vi "configureHWIO_3_statusBusy.vi"(0 "Camera in":refnum<class "Camera.lvclass">, 1 "on":bool=TRUE, 2 "polarity":u16(ring)=1 items=["high level"=1, "low level"=2], 3 "signal_type":u32(ring) items=["Status Busy", "Status Expos", "Status Line", "Status Armed"], 5 "error in (no error)":errorcluster) -> (14 "Camera out":refnum<class "Camera.lvclass">, 19 "error out":errorcluster)   [LabVIEW 2019, in "Camera.lvclass"]
doc: "Configures HWIO 3 status busy for polarity and status (enabled / disabled), and also fuction (exposure or line). Generates an error if camera is recording or if HWIO configuration is not supported."
uses:
  Camera.lvclass
  pco.sdk/CameraDescription/CameraDescription.lvlib
  pco.sdk/TimingControl/TimingControl.lvlib
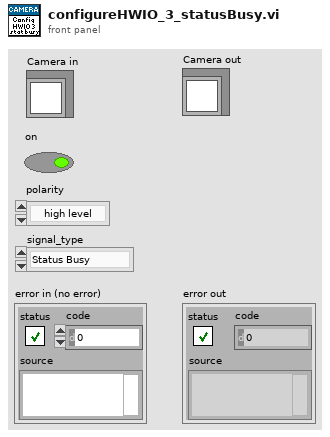
[diagram p1: front panel]
types:
  T1 = cluster{"wSensorTypeDESC":u16, "wSensorSubTypeDESC":u16, "wMaxHorzResStdDESC":u16, "wMaxVertResStdDESC":u16, "wMaxHorzResExtDESC":u16, "wMaxVertResExtDESC":u16, "wDynResDESC":u16, "wMaxBinHorzDESC":u16, "wBinHorzSteppingDESC":u16, "wMaxBinVertDESC":u16, "wBinVertSteppingDESC":u16, "wRoiHorStepsDESC":u16, "wRoiVertStepsDESC":u16, "wNumADCsDESC":u16, "wMinSizeHorzDESC":u16, "dwPixelRateDESC":u32[], "wConvFactDESC":u16[], "sCoolingSetpoints":i16[], "wSoftRoiHorStepsDESC":u16, "wSoftRoiVertStepsDESC":u16, "wIRDESC":u16, "wMinSizeVertDESC":u16, "dwMinDelayDESC":u32, "dwMaxDelayDESC":u32, "dwMinDelayStepDESC":u32, "dwMinExposureDESC":u32, "dwMaxExposureDESC":u32, "dwMinExposureStepDESC":u32, "dwMinDelayIRDESC":u32, "dwMaxDelayIRDESC":u32, "dwMinExposureIRDESC":u32, "dwMaxExposureIRDESC":u32, "wTimeTableDESC":u16, "wDoubleImageDESC":u16, "sMinCoolSetDESC":i16, "sMaxCoolSetDESC":i16, "sDefaultCoolSetDESC":i16, "wPowerDownModeDESC":u16, "wOffsetRegulationDESC":u16, "wColorPatternDESC":u16, "wPatternTypeDESC":u16, "wNumCoolingSetpoints":u16, "dwGeneralCapsDESC1":u32, "dwGeneralCapsDESC2":u32, "dwExtSyncFrequency":u32[], "dwGeneralCapsDESC3":u32, "dwGeneralCapsDESC4":u32}
  T2 = cluster{"wSignalNum":u16, "wEnabled":u16, "wType":u16, "wPolarity":u16, "wFilterSetting":u16, "wSelected":u16, "dwParameter":u32[], "dwSignalFunctionality":u32[]}
  T3 = cluster{"strSignalName":string[], "wSignalDefinitions":u16, "wSignalTypes":u16, "wSignalPolarity":u16, "wSignalFilter":u16}
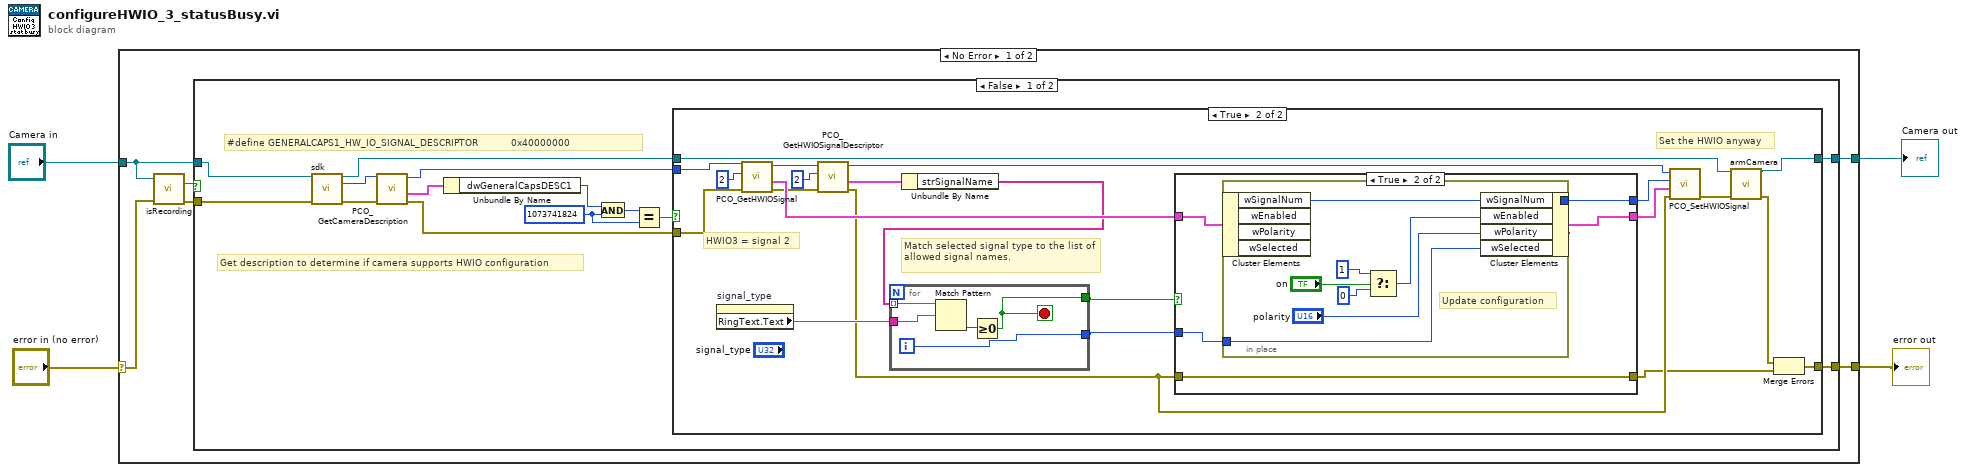
[diagram p0: block diagram]
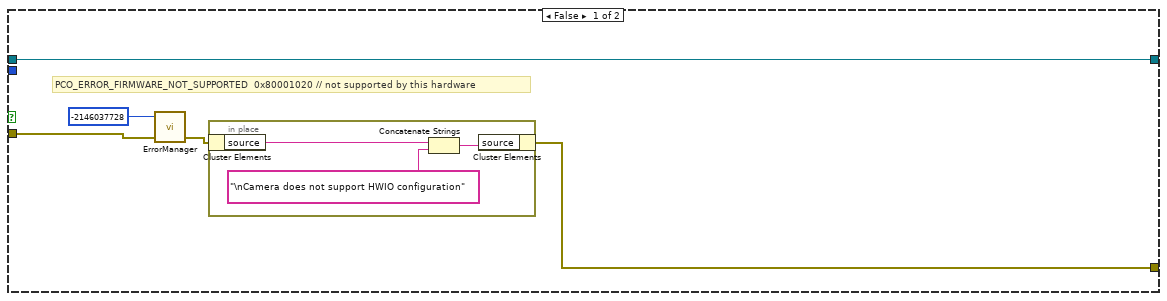
[diagram p2: hidden frame]
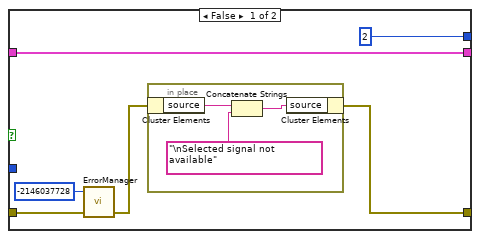
[diagram p3: hidden frame]
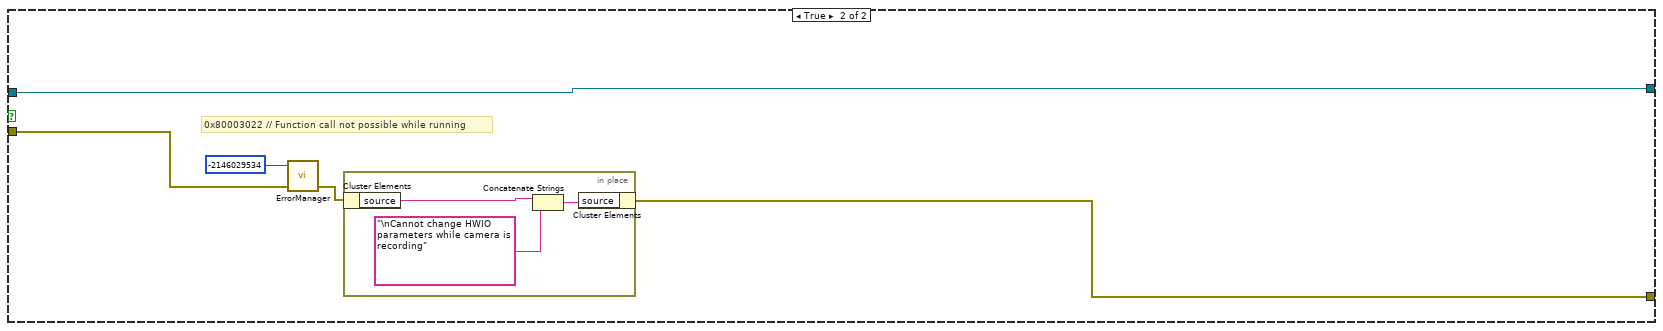
[diagram p4: hidden frame]
diagram:
  n1 = case shown="No Error" "error in (no error)" {
    selector: "error in (no error)" -> [w6 w90]
    tunnel: [w8 w90] -> w3
    tunnel: "Camera in" -> [w10 w89]
    tunnel: [w7 w89] -> w1
    frame No Error {
      n2 = call-dynamic "isRecording.vi"("Camera in"=w10, "error in (no error)"=w6) -> ("recording"=w9:bool, "error out"=w5:errorcluster)  [unwired: 11 in, 1 out]
      n3 = case shown="False" w9 {
        tunnel: w10 -> [w24 w81]
        tunnel: w5 -> [w12 w84]
        tunnel: [w15 w82] -> w8
        tunnel: [w14 w81] -> w7
        frame False {
          w19 = u32 1073741824 ("y")
          # "Get description to determine if camera supports HWIO configuration"
          # "#define GENERALCAPS1_HW_IO_SIGNAL_DESCRIPTOR           0x40000000"
          n4 = call-dynamic "sdk.vi"("Camera in"=w24, "error in (no error)"=w12) -> ("Camera out"=w16:refnum<class "Camera.lvclass">, "sdk"=w23:u64, "error out"=w13:errorcluster)  [unwired: 11 in]
          n5 = call "PCO_GetCameraDescription.vi"("error in (no error)"=w13, "ph"=w23) -> ("error out"=w11:errorcluster, "strDescription"=w22:T1, "ph out"=w17:u64)  [unwired: 6 in, 1 out]
          n6 = Unbundle By Name(w22) -> ("dwGeneralCapsDESC1"=w21:u32)
          n7 = And(x=w21, y=w19) -> (x .and. y?=w20:u32)
          n8 = Equal?(x=w20, y=w19) -> (x = y?=w18:bool)
          n9 = case shown="True" w18 {
            tunnel: w11 -> [w29 w52]
            tunnel: [w26 w36] -> w15
            tunnel: w17 -> [_ w54]
            tunnel: w16 -> [w25 w34]
            tunnel: [w25 w33] -> w14
            frame False {
              # "PCO_ERROR_FIRMWARE_NOT_SUPPORTED  0x80001020 // not supported by this hardware"
              n10 = call "ErrorManager.vi"("error in (no error)"=w29, "error code"=-2146037728) -> ("error out"=w27:errorcluster)  [unwired: 2 in, 1 out]
              n11 = in-place {
                n12 = in-place-cluster #1(w27) -> ("source"=w32:string)
                n13 = Concatenate Strings(w32, "\nCamera does not support HWIO configuration") -> (w30:string)
                n14 = in-place-cluster #1("source"=w30) -> (w26:errorcluster)
              }
            }
            frame True {
              # "Set the HWIO anyway"
              # "Match selected signal type to the list of allowed signal names."
              # "HWIO3 = signal 2"
              n15 = property on="signal_type" class="Ring (strict)"() -> ("RingText.Text"=w41:string)  [unwired: 2 in, 2 out]
              n16 = call "PCO_GetHWIOSignal.vi"("error in (no error)"=w52, "wSignalNum"=u16 2, "ph"=w54) -> ("error out"=w47:errorcluster, "strSignal"=w51:T2, "ph out"=w46:u64)  [unwired: 5 in, 1 out]
              n17 = call "PCO_GetHWIOSignalDescriptor.vi"("error in (no error)"=w47, "wSignalNum"=u16 2, "ph"=w46) -> ("error out"=w38:errorcluster, "strSignalDesc"=w43:T3, "ph out"=w45:u64)  [unwired: 5 in, 1 out]
              n18 = Unbundle By Name(w43) -> ("strSignalName"=w42:string[])
              n19 = for {
                tunnel: w42 -> [w80] mode=indexing
                tunnel: [w77] -> w39
                tunnel: [w76] -> w40
                tunnel: w41 -> [w78]
                i -> [w77]
                stop <- w76 stop-if-true
                n20 = Match Pattern(string=w80, regular expression=w78) -> (offset past match=w79:i32)  [unwired: 1 in, 3 out]
                n21 = Greater Or Equal To 0?(x=w79) -> (x >= 0?=w76:bool)
              }
              n22 = case shown="True" w40 {
                tunnel: w51 -> [w60 w68]
                tunnel: [u16 2 ("wSignalNum") w67] -> w50
                tunnel: [w60 w66] -> w49
                tunnel: w38 -> [w58 w64]
                tunnel: [w55 w64] -> w35
                tunnel: w39 -> [_ w65]
                frame False {
                  n23 = call "ErrorManager.vi"("error in (no error)"=w58, "error code"=-2146037728) -> ("error out"=w56:errorcluster)  [unwired: 2 in, 1 out]
                  n24 = in-place {
                    n25 = in-place-cluster #2(w56) -> ("source"=w63:string)
                    n26 = Concatenate Strings(w63, "\nSelected signal not available" ("string")) -> (w62:string)
                    n27 = in-place-cluster #2("source"=w62) -> (w55:errorcluster)
                  }
                }
                frame True {
                  n28 = in-place {
                    in-place-border: [w70] -> w67
                    in-place-border: w65 -> [w69]
                    # "Update configuration"
                    n29 = in-place-cluster #3(w68) -> ("wSignalNum"=w70:u16)  [unwired: 3 out]
                    n30 = Select(t=u16 1 ("wEnabled"), s="on", f=u16 0 ("wEnabled")) -> (s? t:f=w73:u16)
                    n31 = in-place-cluster #3("wSignalNum"=w70, "wEnabled"=w73, "wPolarity"="polarity", "wSelected"=w69) -> (w66:T2)
                  }
                }
              }
              n32 = call "PCO_SetHWIOSignal.vi"("error in (no error)"=w38, "strSignal"=w49, "wSignalNum"=w50, "ph"=w45) -> ("error out"=w48:errorcluster)  [unwired: 5 in, 2 out]
              n33 = call-dynamic "armCamera.vi"("Camera in"=w34, "error in (no error)"=w48) -> ("Camera out"=w33:refnum<class "Camera.lvclass">, "error out"=w37:errorcluster)  [unwired: 12 in]
              n34 = Merge Errors(w37, w35) -> (w36:errorcluster)
            }
          }
        }
        frame True {
          # "0x80003022 // Function call not possible while running"
          n35 = call "ErrorManager.vi"("error in (no error)"=w84, "error code"=-2146029534) -> ("error out"=w83:errorcluster)  [unwired: 2 in, 1 out]
          n36 = in-place {
            n37 = in-place-cluster #4(w83) -> ("source"=w88:string)
            n38 = Concatenate Strings(w88, "\nCannot change HWIO parameters while camera is recording") -> (w86:string)
            n39 = in-place-cluster #4("source"=w86) -> (w82:errorcluster)
          }
        }
      }
    }
    frame Error {
    }
  }
  "Camera out" <- w1
  "error out" <- w3
